vi "test.assets.vi"() -> ()   [LabVIEW 2020]
uses:
  4d6bbb32-b094-4bc9-b011-261532a2795a.vi
  Nominal Client/Nominal Client.lvclass
  asset/asset.lvclass
  160f26ca-6056-41be-ae64-6851be05d43d.vi
  Nominal Client/asset.get.vi
panel:
  out "x = y? 2":bool
  out "x = y?":bool
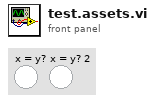
[diagram p1: front panel]
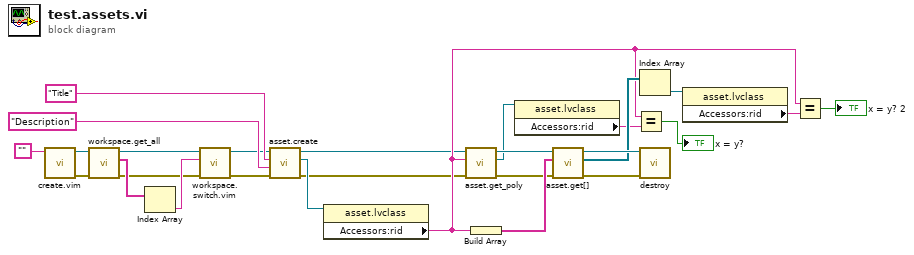
[diagram p0: block diagram]
diagram:
  n1 = call "create.vim"("API Token (string or path)"="") -> ("error out"=w1:errorcluster, "Nominal Client"=w4:refnum<class "Nominal Client.lvclass">)  [unwired: 9 in]
  n2 = call "workspace.get_all.vi"("error in"=w1, "Nominal Client in"=w4) -> ("error out"=w5:errorcluster, "Workspace RIDs"=w8:string[], "Nominal Client out"=w6:refnum<class "Nominal Client.lvclass">)  [unwired: 5 in, 2 out]
  n3 = Index Array(array=w8) -> (element=w7:string)  [unwired: 1 in]
  n4 = call "workspace.switch.vim"("error in"=w5, "Workspace RID (string or path)"=w7, "Nominal Client in"=w6) -> ("error out"=w2:errorcluster, "Nominal Client out"=w3:refnum<class "Nominal Client.lvclass">)  [unwired: 7 in]
  n5 = call "asset.create.vi"("error in"=w2, "Description"="Description", "Title"="Title", "Nominal Client in"=w3) -> ("error out"=w9:errorcluster, "asset"=w24:refnum<class "asset.lvclass">, "Nominal Client out"=w10:refnum<class "Nominal Client.lvclass">)  [unwired: 5 in]
  n6 = property class="asset.lvclass"(reference=w24) -> ("Accessors:rid"=w14:string)  [unwired: 1 in, 2 out]
  n7 = call-poly "asset.get_poly.vi"("error in"=w9, "Asset RID"=w14, "Nominal Client in"=w10) -> ("error out"=w19:errorcluster, "Asset"=w18:refnum<class "asset.lvclass">, "Nominal Client out"=w22:refnum<class "Nominal Client.lvclass">)  [unwired: 6 in]
  n8 = Build Array(w14) -> (w23:string[])
  n9 = property class="asset.lvclass"(reference=w18) -> ("Accessors:rid"=w15:string)  [unwired: 1 in, 2 out]
  n10 = call "asset.get[].vi"("error in"=w19, "Asset RIDs"=w23, "Nominal Client in"=w22) -> ("error out"=w20:errorcluster, "Assets"=w17:refnum<class "asset.lvclass">[], "Nominal Client out"=w21:refnum<class "Nominal Client.lvclass">)  [unwired: 6 in]
  n11 = Equal?(x=w14, y=w15) -> (x = y?=→"x = y?":bool)
  n12 = Index Array(array=w17) -> (element=w16:refnum<class "asset.lvclass">)  [unwired: 1 in]
  n13 = call "destroy.vi"("error in"=w20, "Nominal Client"=w21) -> ()  [unwired: 9 in, 1 out]
  n14 = property class="asset.lvclass"(reference=w16) -> ("Accessors:rid"=w13:string)  [unwired: 1 in, 2 out]
  n15 = Equal?(x=w14, y=w13) -> (x = y?=→"x = y? 2":bool)
